vi "Timed Sequence.vi"() -> ()   [LabVIEW 2015]
uses:
  States.ctl
  <vilib>/eio/EIONode/EIONode.xnode
  <vilib>/rvi/eio/common/nirviEmuTemplateMethod_errors.vi
  <vilib>/platform/TimedLoop/XDataNode/XDataNode.xnode
  <vilib>/Platform/TimedLoop/XDataNode/nitl_modes.ctl
  <vilib>/Platform/TimedLoop/XDataNode/XDNodeRunTimeDep.lvlib
  <vilib>/Platform/TimedLoop/XDataNode/wakeup.ctl
  <vilib>/Platform/TimedLoop/XDataNode/timing_clust.ctl
panel:
  in  "State":T1
  in  "Data":u32=128
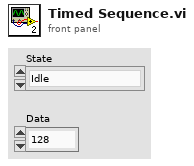
[diagram p1: front panel]
types:
  T1 = typedef "States.ctl" = enum16{"Idle", "CS", "Ready", "Clock High", "Clock Low", "Wait", "Exit"}
  T2 = typedef "XDNodeRunTimeDep.lvlib/timing_clust.ctl" = cluster{"Expected End [f-1]":u64, "Actual End [f-1]":u64, "Finished Late? [f-1]":bool, "Expected End [i-1]":u64, "Actual End [i-1]":u64, "Finished Late? [i-1]":bool, "Expected Start [i]":u64, "Actual Start [i]":u64, "Expected Start [f]":u64, "Actual Start [f]":u64, "Source Name":string, "Structure Name":string, "Period":i64, "Deadline":i64, "Offset":i64, "Start":i64, "Priority":i32, "Timeout":i32, "Mode":T3, "Wakeup Reason":T4, "Error":errorcluster, "Source Type":string, "Secondary Source Type":string, "Global End Time":u64, "Global Start Time":u64, "Frame Duration":u64, "Iteration Duration":u64, "Assigned CPU":i32, "I/O Scan Engine Mode":u32}
  T3 = typedef "XDNodeRunTimeDep.lvlib/nitl_modes.ctl" = enum32{"No Change", "Process missed periods, maintain original phase", "Discard missed periods, maintain original phase", "Process missed periods, ignore original phase", "Discard missed periods, ignore original phase"}
  T4 = typedef "XDNodeRunTimeDep.lvlib/wakeup.ctl" = enum32{"Normal", "Aborted", "Asynchronous wakeup", "Timing source error", "Timed loop error", "Timeout"}
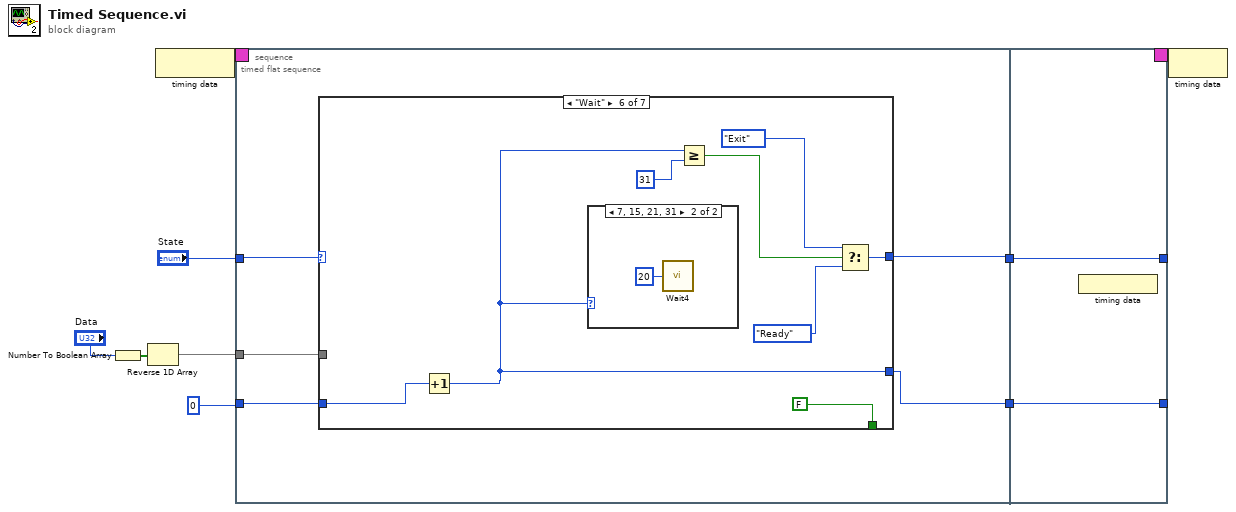
[diagram p0: block diagram]
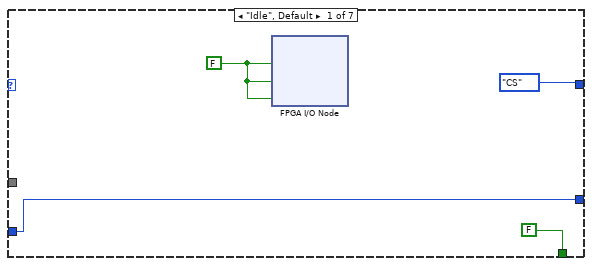
[diagram p2: hidden frame]
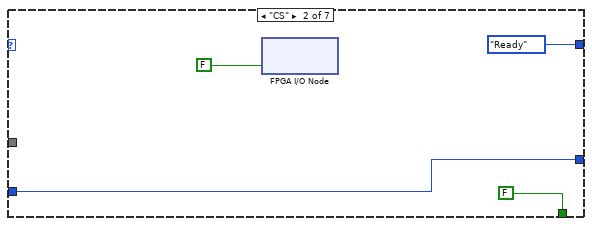
[diagram p3: hidden frame]
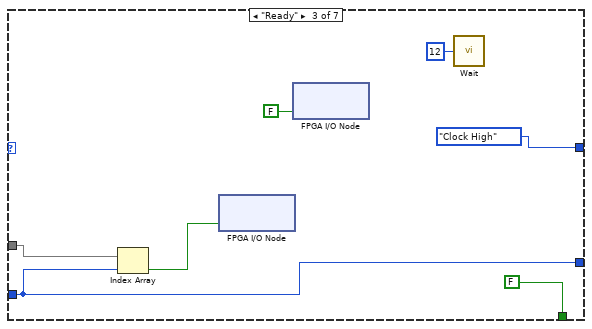
[diagram p4: hidden frame]
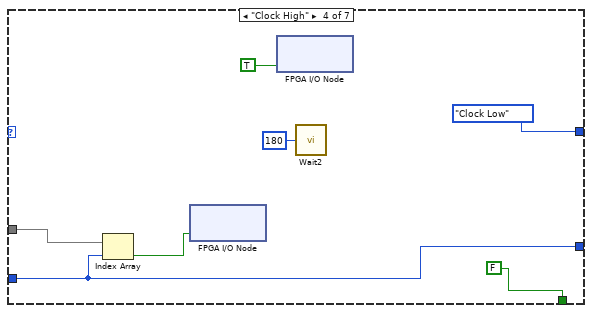
[diagram p5: hidden frame]
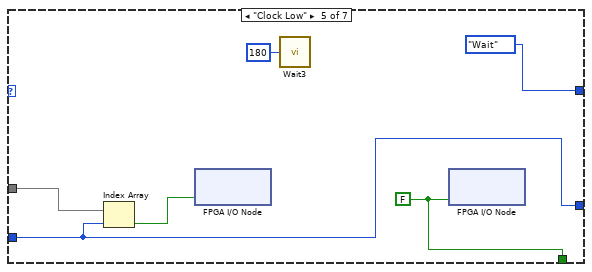
[diagram p6: hidden frame]
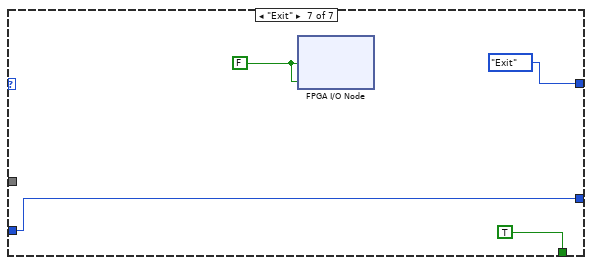
[diagram p8: hidden frame]
diagram:
  n1 = Number To Boolean Array(number="Data") -> (Boolean array=w6:bool[])
  n2 = Reverse 1D Array(array=w6) -> (reversed array=w4:bool[])
  n3 = node-c288() -> (w2:T2)
  n4 = timed-sequence {
    timing: w2 -> [_]
    timing-out: [_] -> w1
    tunnel: w4 -> [w14]
    tunnel: "State" -> [w13]
    tunnel: [w12] -> _
    tunnel: i16 0 -> [w11]
    tunnel: [w10] -> _
    n5 = timed-flat-sequence {
      tunnel: w14 -> [w17]
      tunnel: w13 -> [w19]
      tunnel: w11 -> [w16]
      tunnel: [w18] -> w9
      tunnel: [w15] -> w8
      tunnel: [w63] -> w10
      tunnel: [w64] -> w12
      tunnel: w9 -> [w64]
      tunnel: w8 -> [w63]
      frame #0 {
        n6 = case shown="\"Wait\"" w19 {
          tunnel: [FALSE FALSE FALSE FALSE w47 FALSE TRUE] -> _
          tunnel: [States."CS" ("State") States."Ready" ("State") States."Clock High" ("State") States."Clock Low" ("State") States."Wait" ("State") w51 States."Exit" ("State")] -> w18
          tunnel: w17 -> [_ _ w31 w38 w45 _ _]
          tunnel: w16 -> [w20 w24 w29 w36 w43 w49 w57]
          tunnel: [w20 w24 w29 w36 w43 w48 w57] -> w15
          frame "Idle", Default {
            w21 = FALSE
            n7 = xnode "FPGA I/O Node"("CS"=w21, "SCLK"=w21, "MOSI"=w21) -> ()  [unwired: 3 in, 3 out]
          }
          frame "CS" {
            n8 = xnode "FPGA I/O Node"("CS"=FALSE) -> ()  [unwired: 1 in, 1 out]
          }
          frame "Ready" {
            n9 = Index Array(array=w31, index=w29) -> (element=w30:bool)
            n10 = xnode "FPGA I/O Node"("MOSI"=w30) -> ()  [unwired: 1 in, 1 out]
            n11 = xnode "FPGA I/O Node"("SCLK"=FALSE) -> ()  [unwired: 1 in, 1 out]
            n12 = call "Wait"("Count(Ticks)"=u8 12) -> ()  [unwired: 1 out]
          }
          frame "Clock High" {
            n13 = Index Array(array=w38, index=w36) -> (element=w37:bool)
            n14 = xnode "FPGA I/O Node"("MOSI"=w37) -> ()  [unwired: 1 in, 1 out]
            n15 = xnode "FPGA I/O Node"("SCLK"=TRUE) -> ()  [unwired: 1 in, 1 out]
            n16 = call "Wait2"("Count(Ticks)"=u8 180) -> ()  [unwired: 1 out]
          }
          frame "Clock Low" {
            w47 = FALSE
            n17 = Index Array(array=w45, index=w43) -> (element=w44:bool)
            n18 = xnode "FPGA I/O Node"("MOSI"=w44) -> ()  [unwired: 1 in, 1 out]
            n19 = call "Wait3"("Count(Ticks)"=u8 180) -> ()  [unwired: 1 out]
            n20 = xnode "FPGA I/O Node"("SCLK"=w47) -> ()  [unwired: 1 in, 1 out]
          }
          frame "Wait" {
            n21 = Increment(x=w49) -> (x+1=w48:i16)
            n22 = case shown="7, 15, 21, 31" w48 {
              frame 0, Default {
              }
              frame 7, 15, 21, 31 {
                n23 = call "Wait4"("Count(Ticks)"=u8 20) -> ()  [unwired: 1 out]
              }
            }
            n24 = Greater Or Equal?(x=w48, y=31 ("x")) -> (x >= y?=w54:bool)
            n25 = Select(t=States."Exit" ("State"), s=w54, f=States."Ready" ("State")) -> (s? t:f=w51:T1)
          }
          frame "Exit" {
            w59 = FALSE
            n26 = xnode "FPGA I/O Node"("CS"=w59, "SCLK"=w59) -> ()  [unwired: 2 in, 2 out]
          }
        }
      }
      frame #1 {
        n27 = node-c288() -> ()  [unwired: 1 out]
      }
    }
  }
  n28 = node-c288(w1) -> ()
